vi "Load Active Output Limit Tables.vi"() -> ()   [LabVIEW 2010]
doc: "This function is an offline tool for importing MICS Command and Response Tables from Excel. \n\nInstructions\n1) Copy clipboard from Excel to Import Control.\n2) Run VI.\n3) Edit - Make Current Values Defaults.\n4) Save VI.\n5) Copy tables to new VIs."
panel:
  in  "Table 2":string[][](table)=[["TC7", "Stimulus Phase Amplitude", "", "-5.170", "-4.83", "mA", "GELE"], ["TC7", "Stimulus Phase Pulse Width", "", "7.52", "16.48", "us", "GELE"], ["TC7", "Active Interphase Delay", "", "13", "27", "us", "GELE"], ["TC7", "Active Recovery Phase Amplitude", "", "4.830", "5.145", "mA", "GELE"], ["TC7", "Active Recovery Phase Pulse Width", "", "-13.00", "37.00", "us", "GELE"], ["TC7", "Frequency", "", "1930.0", "2070.0", "Hz", "GELE"], ["TC7", "Pulse Period Jitter (RMS)", "", "-2.50", "2.50", "us", "GELE"], ["TC8", "Stimulus Phase Amplitude", "", "-0.125", "0.085", "mA", "GELE"], ["TC8", "Stimulus Phase Pulse Width", "", "1436", "1564", "us", "GELE"], ["TC8", "Active Interphase Delay", "", "233", "247", "us", "GELE"], ["TC8", "Active Recovery Phase Amplitude", "", "-0.100", "0.115", "mA", "GELE"], ["TC8", "Active Recovery Phase Pulse Width", "", "1,475", "1,525", "us", "GELE"], ["TC8", "Frequency", "", "21.230", "22.770", "Hz", "GELE"], ["TC8", "Pulse Period Jitter (RMS)", "", "-227", "227", "us", "GELE"], ["TC9", "Stimulus Phase Amplitude", "", "-15.320", "-14.68", "mA", "GELE"], ["TC9", "Stimulus Phase Pulse Width", "", "380.00", "420.00", "us", "GELE"], ["TC9", "Active Interphase Delay", "", "93", "107", "us", "GELE"], ["TC9", "Active Recovery Phase Amplitude", "", "14.680", "15.295", "mA", "GELE"], ["TC9", "Active Recovery Phase Pulse Width", "", "375", "425", "us", "GELE"], ["TC9", "Frequency", "", "1.930", "2.070", "Hz", "GELE"], ["TC9", "Pulse Period Jitter (RMS)", "", "-2500", "2500", "us", "GELE"], ["TC10", "Stimulus Phase Amplitude", "", "2.910", "3.09", "mA", "GELE"], ["TC10", "Stimulus Phase Pulse Width", "", "7.52", "16.48", "us", "GELE"], ["TC10", "Active Interphase Delay", "", "13", "27", "us", "GELE"], ["TC10", "Active Recovery Phase Amplitude", "", "-3.150", "-2.875", "mA", "GELE"], ["TC10", "Active Recovery Phase Pulse Width", "", "-13", "37", "us", "GELE"], ["TC10", "Frequency", "", "1544.0", "1656.0", "Hz", "GELE"], ["TC10", "Pulse Period Jitter (RMS)", "", "-3.13", "3.13", "us", "GELE"], ["TC11", "Stimulus Phase Amplitude", "", "-0.085", "0.125", "mA", "GELE"], ["TC11", "Stimulus Phase Pulse Width", "", "1436", "1564", "us", "GELE"], ["TC11", "Active Interphase Delay", "", "233", "247", "us", "GELE"], ["TC11", "Active Recovery Phase Amplitude", "", "-0.140", "0.075", "mA", "GELE"], ["TC11", "Active Recovery Phase Pulse Width", "", "1,475", "1,525", "us", "GELE"], ["TC11", "Frequency", "", "21.230", "22.770", "Hz", "GELE"], ["TC11", "Pulse Period Jitter (RMS)", "", "-227", "227", "us", "GELE"], ["TC11", "Stimulus Phase Amplitude", "", "15.280", "14.720", "mA", "GELE"], ["TC11", "Stimulus Phase Pulse Width", "", "1436", "1564", "us", "GELE"], ["TC11", "Active Interphase Delay", "", "93", "107", "us", "GELE"], ["TC11", "Active Recovery Phase Amplitude", "", "-3.150", "-2.875", "mA", "GELE"], ["TC11", "Active Recovery Phase Pulse Width", "", "7475", "7525", "us", "GELE"], ["TC11", "Frequency", "", "1.930", "2.070", "Hz", "GELE"], ["TC11", "Pulse Period Jitter (RMS)", "", "-2500", "2500", "us", "GELE"]] caption="Table 1"
  out "error out":errorcluster
  in  "error in":errorcluster
  in  "Excel Clipboard to Import 2":string="TC7\tStimulus Phase Amplitude\t-5.170\t-4.83\tmA\tGELE\nTC7\tStimulus Phase Pulse Width\t7.52\t16.48\tus\tGELE\nTC7\tActive Interphase Delay\t13\t27\tus\tGELE\nTC7\tActive Recovery Phase Amplitude\t4.830\t5.145\tmA\tGELE\nTC7\tActive Recovery Phase Pulse Width\t-13.00\t37.00\tus\tGELE\nTC7\tFrequency\t1930.0\t2070.0\tHz\tGELE\nTC7\tPulse Period Jitter (RMS)\t-2.50\t2.50\tus\tGELE\nTC8\tStimulus Phase Amplitude\t-0.125\t0.085\tmA\tGELE\nTC8\tStimulus Phase Pulse Width\t1436\t1564\tus\tGELE\nTC8\tActive Interphase Delay\t233\t247\tus\tGELE\nTC8\tActive Recovery Phase Amplitude\t-0.100\t0.115\tmA\tGELE\nTC8\tActive Recovery Phase Pulse Width\t1,475\t1,525\tus\tGELE\nTC8\tFrequency\t21.230\t22.770\tHz\tGELE\nTC8\tPulse Period Jitter (RMS)\t-227\t227\tus\tGELE\nTC9\tStimulus Phase Amplitude\t-15.320\t-14.68\tmA\tGELE\nTC9\tStimulus Phase Pulse Width\t380.00\t420.00\tus\tGELE\nTC9\tActive Interphase Delay\t93\t107\tus\tGELE\nTC9\tActive Recovery Phase Amplitude\t14.680\t15.295\tmA\tGELE\nTC9\tActive Recovery Phase Pulse Width\t375\t425\tus\tGELE\nTC9\tFrequency\t1.930\t2.070\tHz\tGELE\nTC9\tPulse Period Jitter (RMS)\t-2500\t2500\tus\tGELE\nTC10\tStimulus Phase Amplitude\t2.910\t3.09\tmA\tGELE\nTC10\tStimulus Phase Pulse Width\t7.52\t16.48\tus\tGELE\nTC10\tActive Interphase Delay\t13\t27\tus\tGELE\nTC10\tActive Recovery Phase Amplitude\t-3.150\t-2.875\tmA\tGELE\nTC10\tActive Recovery Phase Pulse Width\t-13\t37\tus\tGELE\nTC10\tFrequency\t1544.0\t1656.0\tHz\tGELE\nTC10\tPulse Period Jitter (RMS)\t-3.13\t3.13\tus\tGELE\nTC11\tStimulus Phase Amplitude\t-0.085\t0.125\tmA\tGELE\nTC11\tStimulus Phase Pulse Width\t1436\t1564\tus\tGELE\nTC11\tActive Interphase Delay\t233\t247\tus\tGELE\nTC11\tActive Recovery Phase Amplitude\t-0.140\t0.075\tmA\tGELE\nTC11\tActive Recovery Phase Pulse Width\t1,475\t1,525\tus\tGELE\nTC11\tFrequency\t21.230\t22.770\tHz\tGELE\nTC11\tPulse Period Jitter (RMS)\t-227\t227\tus\tGELE\nTC11\tStimulus Phase Amplitude\t15.280\t14.720\tmA\tGELE\nTC11\tStimulus Phase Pulse Width\t1436\t1564\tus\tGELE\nTC11\tActive Interphase Delay\t93\t107\tus\tGELE\nTC11\tActive Recovery Phase Amplitude\t-3.150\t-2.875\tmA\tGELE\nTC11\tActive Recovery Phase Pulse Width\t7475\t7525\tus\tGELE\nTC11\tFrequency\t1.930\t2.070\tHz\tGELE\nTC11\tPulse Period Jitter (RMS)\t-2500\t2500\tus\tGELE\n"
  in  "Excel Clipboard1 to Import 1":string="TC1\tStimulus Phase Amplitude\t-5.170\t-4.83\tmA\tGELE\nTC1\tStimulus Phase Pulse Width\t7.52\t16.48\tus\tGELE\nTC1\tActive Interphase Delay\t13\t27\tus\tGELE\nTC1\tActive Recovery Phase Amplitude\t4.830\t5.145\tmA\tGELE\nTC1\tActive Recovery Phase Pulse Width\t-13.00\t37.00\tus\tGELE\nTC1\tFrequency\t1930.0\t2070.0\tHz\tGELE\nTC1\tPulse Period Jitter (RMS)\t-2.50\t2.50\tus\tGELE\nTC2\tStimulus Phase Amplitude\t-0.125\t0.085\tmA\tGELE\nTC2\tStimulus Phase Pulse Width\t1436\t1564\tus\tGELE\nTC2\tActive Interphase Delay\t233\t247\tus\tGELE\nTC2\tActive Recovery Phase Amplitude\t-0.100\t0.115\tmA\tGELE\nTC2\tActive Recovery Phase Pulse Width\t1,475\t1,525\tus\tGELE\nTC2\tFrequency\t21.230\t22.770\tHz\tGELE\nTC2\tPulse Period Jitter (RMS)\t-227\t227\tus\tGELE\nTC3\tStimulus Phase Amplitude\t-15.320\t-14.68\tmA\tGELE\nTC3\tStimulus Phase Pulse Width\t380.00\t420.00\tus\tGELE\nTC3\tActive Interphase Delay\t93\t107\tus\tGELE\nTC3\tActive Recovery Phase Amplitude\t14.680\t15.295\tmA\tGELE\nTC3\tActive Recovery Phase Pulse Width\t375\t425\tus\tGELE\nTC3\tFrequency\t1.930\t2.070\tHz\tGELE\nTC3\tPulse Period Jitter (RMS)\t-2500\t2500\tus\tGELE\nTC4\tStimulus Phase Amplitude\t2.910\t3.09\tmA\tGELE\nTC4\tStimulus Phase Pulse Width\t7.52\t16.48\tus\tGELE\nTC4\tActive Interphase Delay\t13\t27\tus\tGELE\nTC4\tActive Recovery Phase Amplitude\t-3.150\t-2.875\tmA\tGELE\nTC4\tActive Recovery Phase Pulse Width\t-13\t37\tus\tGELE\nTC4\tFrequency\t1544.0\t1656.0\tHz\tGELE\nTC4\tPulse Period Jitter (RMS)\t-3.13\t3.13\tus\tGELE\nTC5\tStimulus Phase Amplitude\t-0.085\t0.125\tmA\tGELE\nTC5\tStimulus Phase Pulse Width\t1436\t1564\tus\tGELE\nTC5\tActive Interphase Delay\t233\t247\tus\tGELE\nTC5\tActive Recovery Phase Amplitude\t-0.140\t0.075\tmA\tGELE\nTC5\tActive Recovery Phase Pulse Width\t1,475\t1,525\tus\tGELE\nTC5\tFrequency\t21.230\t22.770\tHz\tGELE\nTC5\tPulse Period Jitter (RMS)\t-227\t227\tus\tGELE\nTC6\tStimulus Phase Amplitude\t15.280\t14.720\tmA\tGELE\nTC6\tStimulus Phase Pulse Width\t1436\t1564\tus\tGELE\nTC6\tActive Interphase Delay\t93\t107\tus\tGELE\nTC6\tActive Recovery Phase Amplitude\t-3.150\t-2.875\tmA\tGELE\nTC6\tActive Recovery Phase Pulse Width\t7475\t7525\tus\tGELE\nTC6\tFrequency\t1.930\t2.070\tHz\tGELE\nTC6\tPulse Period Jitter (RMS)\t-2500\t2500\tus\tGELE\n"
  in  "Table 1":string[][](table)=[["TC1", "Stimulus Phase Amplitude", "", "-5.170", "-4.83", "mA", "GELE"], ["TC1", "Stimulus Phase Pulse Width", "", "7.52", "16.48", "us", "GELE"], ["TC1", "Active Interphase Delay", "", "13", "27", "us", "GELE"], ["TC1", "Active Recovery Phase Amplitude", "", "4.830", "5.145", "mA", "GELE"], ["TC1", "Active Recovery Phase Pulse Width", "", "-13.00", "37.00", "us", "GELE"], ["TC1", "Frequency", "", "1930.0", "2070.0", "Hz", "GELE"], ["TC1", "Pulse Period Jitter (RMS)", "", "-2.50", "2.50", "us", "GELE"], ["TC2", "Stimulus Phase Amplitude", "", "-0.125", "0.085", "mA", "GELE"], ["TC2", "Stimulus Phase Pulse Width", "", "1436", "1564", "us", "GELE"], ["TC2", "Active Interphase Delay", "", "233", "247", "us", "GELE"], ["TC2", "Active Recovery Phase Amplitude", "", "-0.100", "0.115", "mA", "GELE"], ["TC2", "Active Recovery Phase Pulse Width", "", "1,475", "1,525", "us", "GELE"], ["TC2", "Frequency", "", "21.230", "22.770", "Hz", "GELE"], ["TC2", "Pulse Period Jitter (RMS)", "", "-227", "227", "us", "GELE"], ["TC3", "Stimulus Phase Amplitude", "", "-15.320", "-14.68", "mA", "GELE"], ["TC3", "Stimulus Phase Pulse Width", "", "380.00", "420.00", "us", "GELE"], ["TC3", "Active Interphase Delay", "", "93", "107", "us", "GELE"], ["TC3", "Active Recovery Phase Amplitude", "", "14.680", "15.295", "mA", "GELE"], ["TC3", "Active Recovery Phase Pulse Width", "", "375", "425", "us", "GELE"], ["TC3", "Frequency", "", "1.930", "2.070", "Hz", "GELE"], ["TC3", "Pulse Period Jitter (RMS)", "", "-2500", "2500", "us", "GELE"], ["TC4", "Stimulus Phase Amplitude", "", "2.910", "3.09", "mA", "GELE"], ["TC4", "Stimulus Phase Pulse Width", "", "7.52", "16.48", "us", "GELE"], ["TC4", "Active Interphase Delay", "", "13", "27", "us", "GELE"], ["TC4", "Active Recovery Phase Amplitude", "", "-3.150", "-2.875", "mA", "GELE"], ["TC4", "Active Recovery Phase Pulse Width", "", "-13", "37", "us", "GELE"], ["TC4", "Frequency", "", "1544.0", "1656.0", "Hz", "GELE"], ["TC4", "Pulse Period Jitter (RMS)", "", "-3.13", "3.13", "us", "GELE"], ["TC5", "Stimulus Phase Amplitude", "", "-0.085", "0.125", "mA", "GELE"], ["TC5", "Stimulus Phase Pulse Width", "", "1436", "1564", "us", "GELE"], ["TC5", "Active Interphase Delay", "", "233", "247", "us", "GELE"], ["TC5", "Active Recovery Phase Amplitude", "", "-0.140", "0.075", "mA", "GELE"], ["TC5", "Active Recovery Phase Pulse Width", "", "1,475", "1,525", "us", "GELE"], ["TC5", "Frequency", "", "21.230", "22.770", "Hz", "GELE"], ["TC5", "Pulse Period Jitter (RMS)", "", "-227", "227", "us", "GELE"], ["TC6", "Stimulus Phase Amplitude", "", "15.280", "14.720", "mA", "GELE"], ["TC6", "Stimulus Phase Pulse Width", "", "1436", "1564", "us", "GELE"], ["TC6", "Active Interphase Delay", "", "93", "107", "us", "GELE"], ["TC6", "Active Recovery Phase Amplitude", "", "-3.150", "-2.875", "mA", "GELE"], ["TC6", "Active Recovery Phase Pulse Width", "", "7475", "7525", "us", "GELE"], ["TC6", "Frequency", "", "1.930", "2.070", "Hz", "GELE"], ["TC6", "Pulse Period Jitter (RMS)", "", "-2500", "2500", "us", "GELE"]]
  # "Instructions\n1) Copy clipboard from Excel to Import Control.\n2) Run VI.\n3) Edit - Make Current Values Defaults.\n4) Save VI.\n5) Copy tables to new VIs."
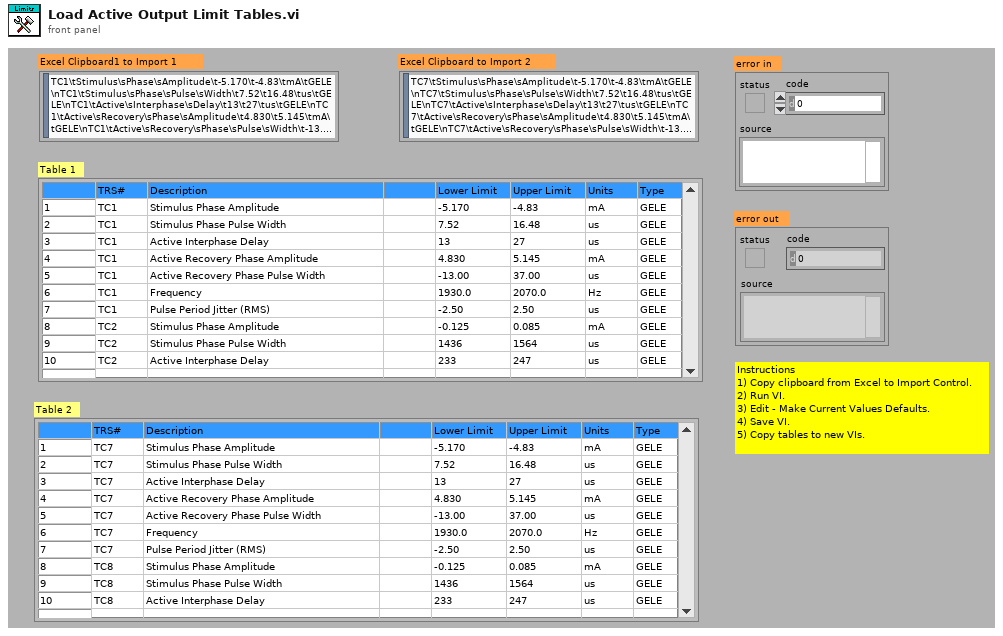
[diagram p1: front panel]
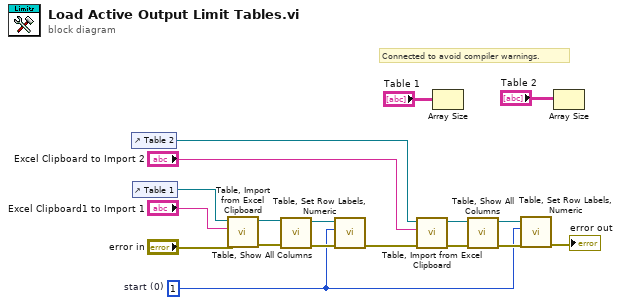
[diagram p0: block diagram]
diagram:
  w5 = 1  # start (0)
  # "Connected to avoid compiler warnings."
  n1 = control-ref of="Table 2"() -> (w1:refnum<vi>)
  n2 = control-ref of="Table 1"() -> (w17:refnum<vi>)
  n3 = call "Table, Import from Excel Clipboard.vi"("error in"="error in", "Excel Clipboard to Import"="Excel Clipboard1 to Import 1", "Tbl Refnum"=w17) -> ("error out"=w15:errorcluster, "Tbl Refnumout"=w16:refnum<vi>)  [unwired: 7 in]
  n4 = call "Table, Show All Columns.vi"("error in"=w15, "Tbl Refnum"=w16) -> ("error out"=w13:errorcluster, "Tbl Refnum out"=w12:refnum<vi>)  [unwired: 8 in]
  n5 = call "Table, Set Row Labels, Numeric.vi"("error in"=w13, "start (0)"=w5, "Tbl Refnum"=w12) -> ("error out"=w11:errorcluster)  [unwired: 7 in, 1 out]
  n6 = call "Table, Import from Excel Clipboard.vi"("error in"=w11, "Excel Clipboard to Import"="Excel Clipboard to Import 2", "Tbl Refnum"=w1) -> ("error out"=w10:errorcluster, "Tbl Refnumout"=w4:refnum<vi>)  [unwired: 7 in]
  n7 = Array Size(array="Table 1") -> ()  [unwired: 1 out]
  n8 = call "Table, Show All Columns.vi"("error in"=w10, "Tbl Refnum"=w4) -> ("error out"=w9:errorcluster, "Tbl Refnum out"=w3:refnum<vi>)  [unwired: 8 in]
  n9 = call "Table, Set Row Labels, Numeric.vi"("error in"=w9, "start (0)"=w5, "Tbl Refnum"=w3) -> ("error out"=→"error out":errorcluster)  [unwired: 7 in, 1 out]
  n10 = Array Size(array="Table 2") -> ()  [unwired: 1 out]
